vi "setPhase.vi"(8 "error in (no error)":errorcluster, 10 "phase":dbl, 11 "SingleTone.lvclass in":refnum<class "SingleTone.lvclass">) -> (0 "error out":errorcluster, 3 "SingleTone.lvclass out":refnum<class "SingleTone.lvclass">)   [LabVIEW 2011, in "Tools.lvlib" / "Scripting.lvlib" / "SingleTone.lvclass"]
uses:
  SingleTone.lvclass
  SingleTone.lvclass/SingleTone.ctl
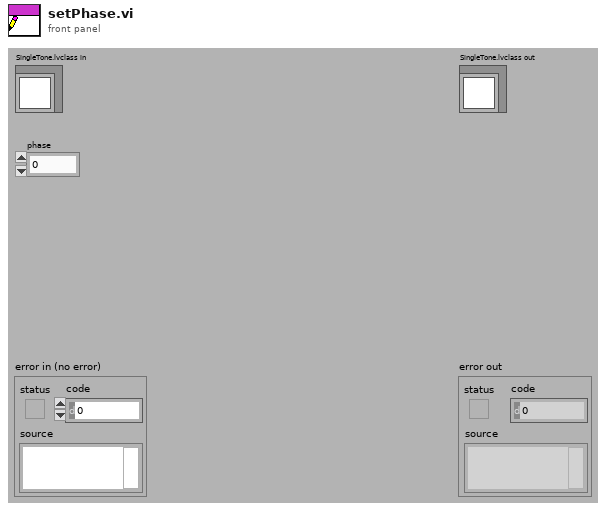
[diagram p1: front panel]
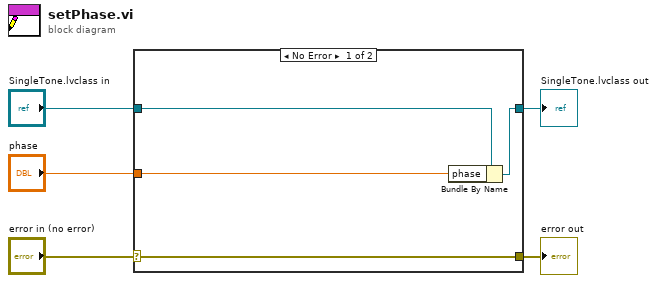
[diagram p0: block diagram]
diagram:
  n1 = case shown="No Error" "error in (no error)" {
    selector: "error in (no error)" -> [w9 w10]
    tunnel: [w9 w10] -> w4
    tunnel: [w7 w11] -> w2
    tunnel: "SingleTone.lvclass in" -> [w8 w11]
    tunnel: "phase" -> [w6 _]
    frame No Error {
      n2 = Bundle By Name(cluster=w8, "phase"=w6) -> (w7:refnum<class "SingleTone.lvclass">)
    }
    frame Error {
    }
  }
  "error out" <- w4
  "SingleTone.lvclass out" <- w2
